vi "instr.DSO2002A.vi"(0 "VISA资源名称":refnum<visa-resource-name>, 1 "CMD":T2(ring), 2 "Trigger Mode":enum16{" TV", " GLITch", " EDGE", " PATTern"}(ring), 3 "Trigger Sweep":enum16{" AUTO", " NORMAL"}(ring), 4 "SignalFreq(kHz)":dbl=1.0, 5 "错误输入（无错误）":errorcluster, 6 "SignalVpp(V)":dbl=5.0, 7 "source":enum16{"  CHANnel1", "  CHANnel2"}(ring), 8 "Polarity":enum16{" NEGative", " POSitive"}(ring), 9 "Acquire Mode":enum16{" SEGMented", " RTIMe"}(ring), 10 "Standard":enum16{" PAL", " NTSC", " PALM", " SECam"}(ring), 11 "Reference":enum16{" CENTer", " LEFT", " RIGHt"}(ring), 13 "Acquire Type":T1(ring)) -> (14 "OK?":bool, 15 "Return Value":dbl, 18 "波形图":u8[](graph), 19 "错误输出":errorcluster)   [LabVIEW 2012, in "Lib_UEL.ATE.lvlib" / "Lib_Instrument.lvlib"]
uses:
  Lib_Instrument.lvlib
panel:
  in  "?":enum32{"TV", "Glitch"}(tab)
  in  "Setting":refnum<k24>(container)
  # "- 初始版本。\n- 2012-12-03: 增加获取图像命令，增加RESET命令。\n              命令子VI开放命令超时设置，默认超时为200mS。\n              留意：RESET命令需要1000mS超时才能正确工作。 \n-2013-5-20:增加触发&获取一部分功能\n-2013-5-21:增加自动获取和交流采集"
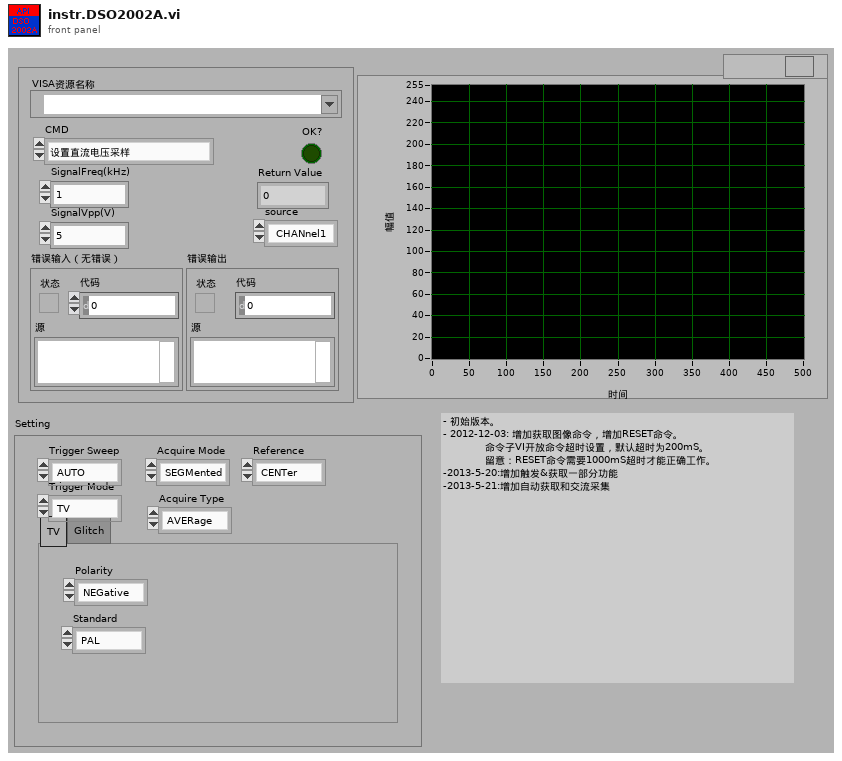
[diagram p1: front panel]
types:
  T1 = enum16{" AVERage", " NORMal", " HRESolution", " PEAK", ""}
  T2 = enum16{"设置直流电压采样", "设置交流电压采样", "获取直流电压值", "设置RMS采样", "获取RMS值", "设置频率采样", "获取频率值", "获取VPP", "重设Timing", "获取波形图", "RESET", "OFFSET", "设置触发模式", "设置获取模式", "自动获取", "Measure Vavg"}
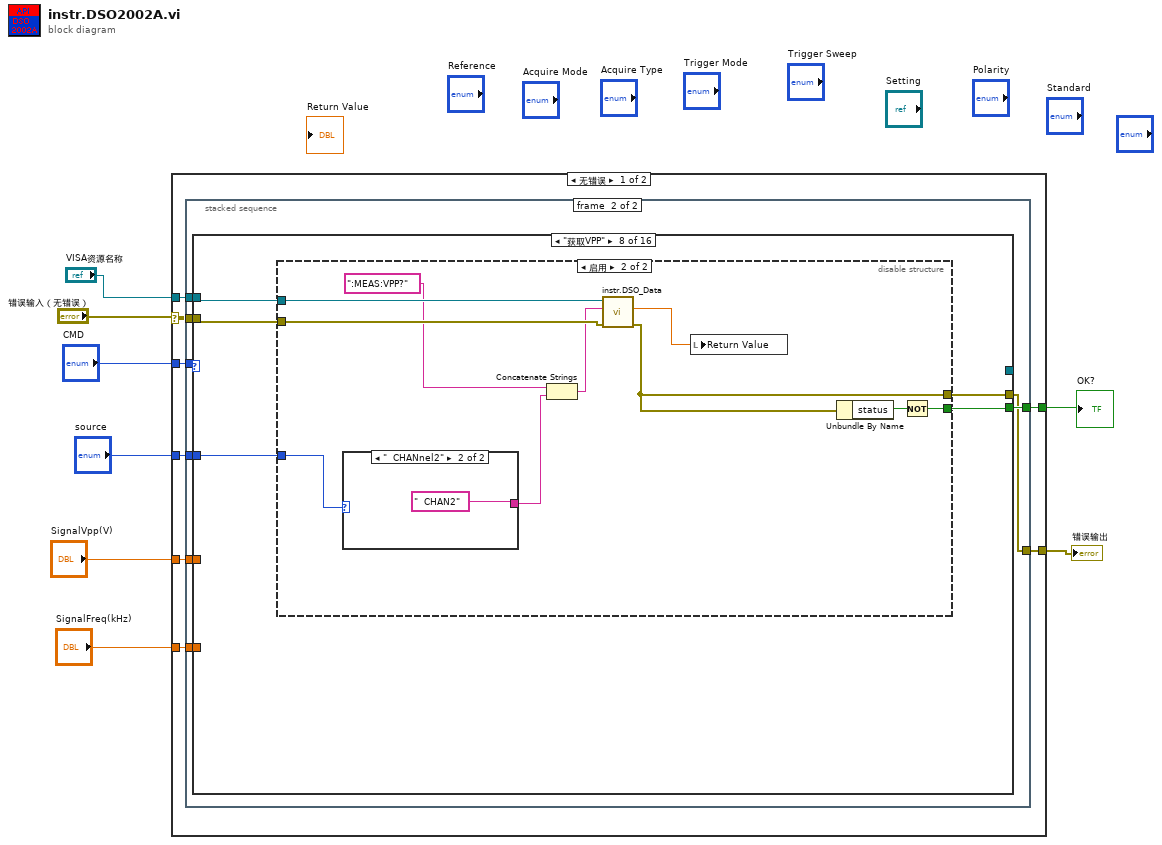
[diagram p0: block diagram]
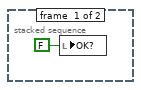
[diagram p2: hidden frame]
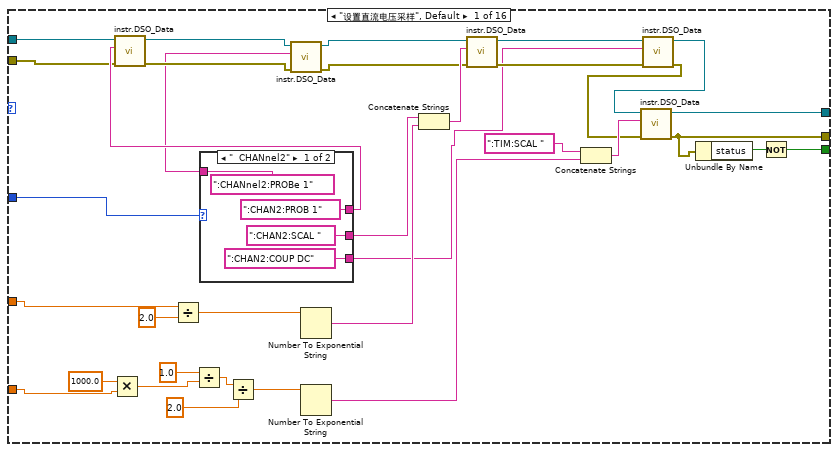
[diagram p3: hidden frame]
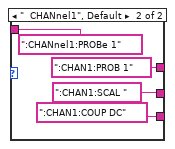
[diagram p4: hidden frame]
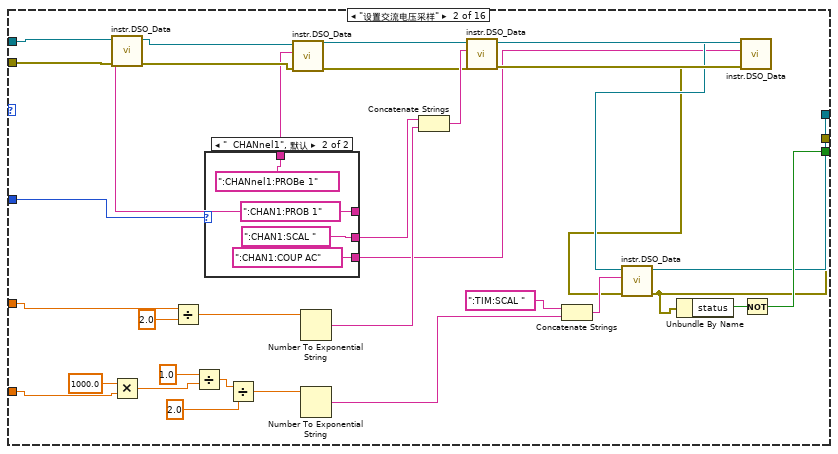
[diagram p5: hidden frame]
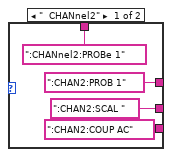
[diagram p6: hidden frame]
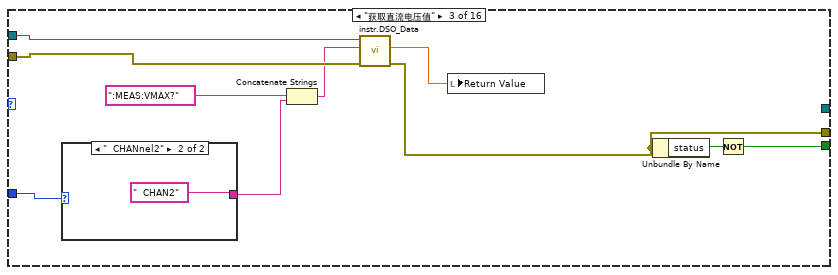
[diagram p7: hidden frame]
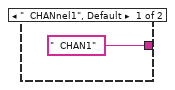
[diagram p8: hidden frame]
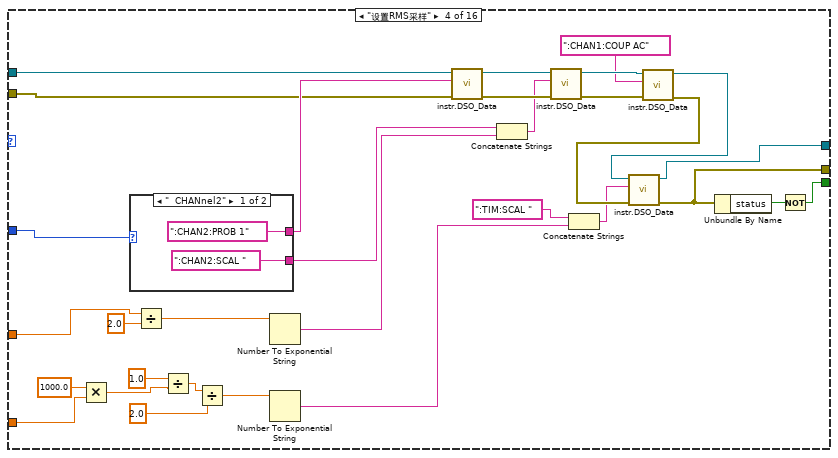
[diagram p9: hidden frame]
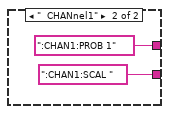
[diagram p10: hidden frame]
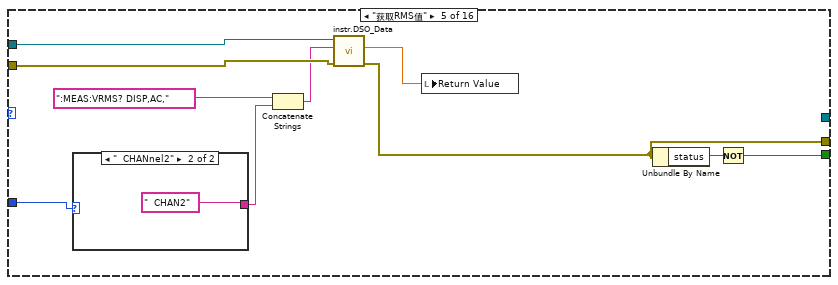
[diagram p11: hidden frame]
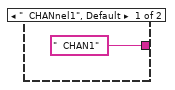
[diagram p12: hidden frame]
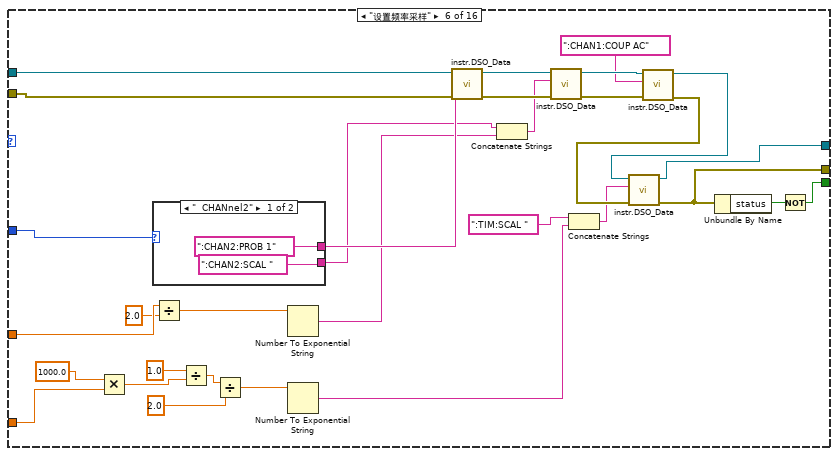
[diagram p13: hidden frame]
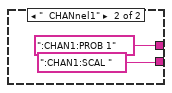
[diagram p14: hidden frame]
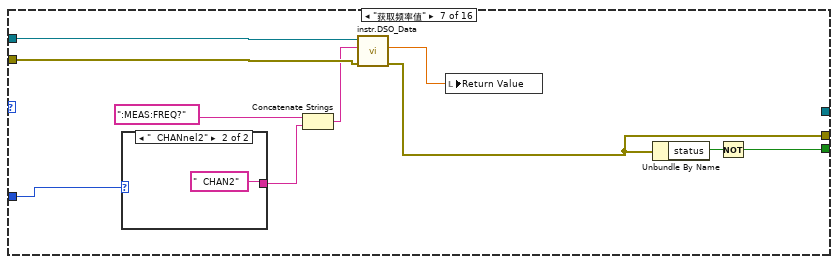
[diagram p15: hidden frame]
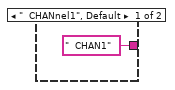
[diagram p16: hidden frame]
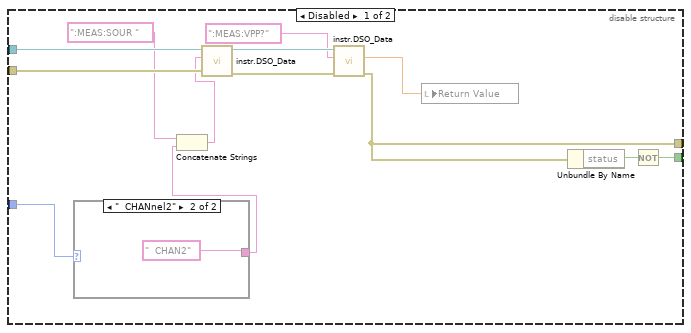
[diagram p17: hidden frame]
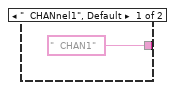
[diagram p18: hidden frame]
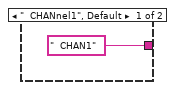
[diagram p19: hidden frame]
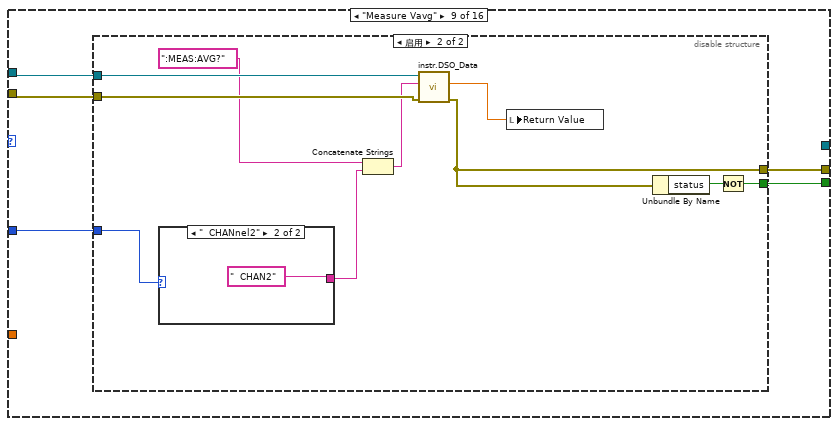
[diagram p20: hidden frame]
diagram:
  n1 = case shown="无错误" "错误输入（无错误）" {
    selector: "错误输入（无错误）" -> [w14 w428]
    tunnel: "VISA资源名称" -> [w16 _]
    tunnel: "CMD" -> [w15 _]
    tunnel: [w13 FALSE] -> w5
    tunnel: "SignalFreq(kHz)" -> [w12 _]
    tunnel: "SignalVpp(V)" -> [w11 _]
    tunnel: [w10 w428] -> w2
    tunnel: "source" -> [w9 _]
    frame No Error {
      n2 = stacked-sequence {
        tunnel: w16 -> [_ w25]
        tunnel: w15 -> [_ w24]
        tunnel: w14 -> [_ w18]
        tunnel: [_ w21] -> w13
        tunnel: w12 -> [_ w23]
        tunnel: w11 -> [_ w22]
        tunnel: [_ w20] -> w10
        tunnel: w9 -> [_ w19]
        frame #0 {
          n3 = local write "OK?"(FALSE ("OK?")) -> ()
        }
        frame #1 {
          n4 = case shown="\"获取VPP\"" w24 {
            tunnel: w25 -> [w34 w74 w119 w123 w166 w170 w213 w220 w252 w283 w306 w322 w361 w373 w420 w426]
            tunnel: [w56 w97 w115 w145 w162 w192 w209 w218 w250 w294 w310 w348 w356 w367 w403 w422] -> w21
            tunnel: w23 -> [w46 w87 _ w141 _ w188 _ _ _ w290 _ _ _ _ _ _]
            tunnel: w22 -> [w47 w88 _ w132 _ w179 _ _ _ _ _ _ _ w365 _ _]
            tunnel: [w38 w79 _ w125 _ w173 _ _ _ w281 w308 w327 w354 w371 w411 w424] -> _
            tunnel: [w37 w78 w114 w126 w161 w174 w208 w217 w249 w280 w307 w317 w353 w366 w402 w421] -> w20
            tunnel: w19 -> [w36 w77 w113 w124 w160 w172 w204 w216 w248 _ w304 _ _ _ _ _]
            tunnel: w18 -> [w33 w71 w118 w122 w165 w169 w212 w219 w251 w282 w305 w321 w360 w377 w419 w425]
            frame "设置直流电压采样", Default {
              n5 = Multiply(x=1000.0, y=w46) -> (x*y=w52:dbl)
              n6 = Divide(x=w47, y=2.0) -> (x/y=w48:dbl)
              n7 = Divide(x=1.0, y=w52) -> (x/y=w54:dbl)
              n8 = case shown="\"  CHANnel2\"" w36 {
                tunnel: [":CHAN2:PROB 1" ("CMD write") ":CHAN1:PROB 1" ("CMD write")] -> w59
                tunnel: [":CHAN2:SCAL " ("CMD write") ":CHAN1:SCAL " ("CMD write")] -> w35
                tunnel: [":CHAN2:COUP DC" ("CMD write") ":CHAN1:COUP DC" ("CMD write")] -> w32
                tunnel: [":CHANnel2:PROBe 1" ("CMD write") ":CHANnel1:PROBe 1" ("CMD write")] -> w26
                frame "  CHANnel2" {
                }
                frame "  CHANnel1", Default {
                }
              }
              n9 = call "instr.DSO_Data.vi"("错误输入（无错误）"=w33, "CMD write"=w59, "VISA.in"=w34) -> ("错误输出"=w28:errorcluster, "VISA.out"=w30:refnum<visa-resource-name>)  [unwired: 5 in, 2 out]
              n10 = Divide(x=w54, y=2.0) -> (x/y=w50:dbl)
              n11 = call "instr.DSO_Data.vi"("错误输入（无错误）"=w28, "CMD write"=w26, "VISA.in"=w30) -> ("错误输出"=w27:errorcluster, "VISA.out"=w29:refnum<visa-resource-name>)  [unwired: 5 in, 2 out]
              n12 = Number To Exponential String(number=w48) -> (E-format string=w40:string)  [unwired: 3 in]
              n13 = Number To Exponential String(number=w50) -> (E-format string=w41:string)  [unwired: 3 in]
              n14 = Concatenate Strings(w35, w40) -> (w39:string)
              n15 = call "instr.DSO_Data.vi"("错误输入（无错误）"=w27, "CMD write"=w39, "VISA.in"=w29) -> ("错误输出"=w58:errorcluster, "VISA.out"=w31:refnum<visa-resource-name>)  [unwired: 5 in, 2 out]
              n16 = Concatenate Strings(":TIM:SCAL " ("CMD write"), w41) -> (w44:string)
              n17 = call "instr.DSO_Data.vi"("错误输入（无错误）"=w58, "CMD write"=w32, "VISA.in"=w31) -> ("错误输出"=w42:errorcluster, "VISA.out"=w43:refnum<visa-resource-name>)  [unwired: 5 in, 2 out]
              n18 = call "instr.DSO_Data.vi"("错误输入（无错误）"=w42, "CMD write"=w44, "VISA.in"=w43) -> ("错误输出"=w37:errorcluster, "VISA.out"=w38:refnum<visa-resource-name>)  [unwired: 5 in, 2 out]
              n19 = Unbundle By Name(w37) -> ("status"=w57:bool)
              n20 = Not(x=w57) -> (.not. x?=w56:bool)
            }
            frame "设置交流电压采样" {
              n21 = Multiply(x=1000.0, y=w87) -> (x*y=w93:dbl)
              n22 = Divide(x=w88, y=2.0) -> (x/y=w89:dbl)
              n23 = Divide(x=1.0, y=w93) -> (x/y=w95:dbl)
              n24 = case shown="\"  CHANnel1\", 默认" w77 {
                tunnel: [":CHAN2:PROB 1" ("CMD write") ":CHAN1:PROB 1" ("CMD write")] -> w101
                tunnel: [":CHAN2:SCAL " ("CMD write") ":CHAN1:SCAL " ("CMD write")] -> w76
                tunnel: [":CHAN2:COUP AC" ("CMD write") ":CHAN1:COUP AC" ("CMD write")] -> w75
                tunnel: [":CHANnel2:PROBe 1" ("CMD write") ":CHANnel1:PROBe 1" ("CMD write")] -> w68
                frame "  CHANnel2" {
                }
                frame "  CHANnel1", Default {
                }
              }
              n25 = call "instr.DSO_Data.vi"("错误输入（无错误）"=w71, "CMD write"=w101, "VISA.in"=w74) -> ("错误输出"=w72:errorcluster, "VISA.out"=w73:refnum<visa-resource-name>)  [unwired: 5 in, 2 out]
              n26 = Divide(x=w95, y=2.0) -> (x/y=w91:dbl)
              n27 = call "instr.DSO_Data.vi"("错误输入（无错误）"=w72, "CMD write"=w68, "VISA.in"=w73) -> ("错误输出"=w70:errorcluster, "VISA.out"=w69:refnum<visa-resource-name>)  [unwired: 5 in, 2 out]
              n28 = Number To Exponential String(number=w89) -> (E-format string=w81:string)  [unwired: 3 in]
              n29 = Number To Exponential String(number=w91) -> (E-format string=w82:string)  [unwired: 3 in]
              n30 = Concatenate Strings(w76, w81) -> (w80:string)
              n31 = call "instr.DSO_Data.vi"("错误输入（无错误）"=w70, "CMD write"=w80, "VISA.in"=w69) -> ("错误输出"=w99:errorcluster, "VISA.out"=w100:refnum<visa-resource-name>)  [unwired: 5 in, 2 out]
              n32 = Concatenate Strings(":TIM:SCAL " ("CMD write"), w82) -> (w85:string)
              n33 = call "instr.DSO_Data.vi"("错误输入（无错误）"=w99, "CMD write"=w75, "VISA.in"=w100) -> ("错误输出"=w83:errorcluster, "VISA.out"=w84:refnum<visa-resource-name>)  [unwired: 5 in, 2 out]
              n34 = call "instr.DSO_Data.vi"("错误输入（无错误）"=w83, "CMD write"=w85, "VISA.in"=w84) -> ("错误输出"=w78:errorcluster, "VISA.out"=w79:refnum<visa-resource-name>)  [unwired: 5 in, 2 out]
              n35 = Unbundle By Name(w78) -> ("status"=w98:bool)
              n36 = Not(x=w98) -> (.not. x?=w97:bool)
            }
            frame "获取直流电压值" {
              n37 = case shown="\"  CHANnel2\"" w113 {
                tunnel: ["  CHAN1" ("CMD write") "  CHAN2" ("CMD write")] -> w111
                frame "  CHANnel1", Default {
                }
                frame "  CHANnel2" {
                }
              }
              n38 = Concatenate Strings(":MEAS:VMAX?" ("CMD write"), w111) -> (w110:string)
              n39 = call "instr.DSO_Data.vi"("错误输入（无错误）"=w118, "CMD write"=w110, "VISA.in"=w119) -> ("错误输出"=w114:errorcluster, "Value"=w117:dbl)  [unwired: 5 in, 2 out]
              n40 = local write "Return Value"(w117) -> ()
              n41 = Unbundle By Name(w114) -> ("status"=w116:bool)
              n42 = Not(x=w116) -> (.not. x?=w115:bool)
            }
            frame "设置RMS采样" {
              n43 = Multiply(x=1000.0, y=w141) -> (x*y=w140:dbl)
              n44 = case shown="\"  CHANnel2\"" w124 {
                tunnel: [":CHAN2:PROB 1" ("CMD write") ":CHAN1:PROB 1" ("CMD write")] -> w152
                tunnel: [":CHAN2:SCAL " ("CMD write") ":CHAN1:SCAL " ("CMD write")] -> w130
                frame "  CHANnel2" {
                }
                frame "  CHANnel1" {
                }
              }
              n45 = Divide(x=w132, y=2.0) -> (x/y=w129:dbl)
              n46 = Divide(x=1.0, y=w140) -> (x/y=w143:dbl)
              n47 = Divide(x=w143, y=2.0) -> (x/y=w138:dbl)
              n48 = Number To Exponential String(number=w129) -> (E-format string=w128:string)  [unwired: 3 in]
              n49 = Number To Exponential String(number=w138) -> (E-format string=w134:string)  [unwired: 3 in]
              n50 = call "instr.DSO_Data.vi"("错误输入（无错误）"=w122, "CMD write"=w152, "VISA.in"=w123) -> ("错误输出"=w150:errorcluster, "VISA.out"=w151:refnum<visa-resource-name>)  [unwired: 5 in, 2 out]
              n51 = Concatenate Strings(w130, w128) -> (w127:string)
              n52 = call "instr.DSO_Data.vi"("错误输入（无错误）"=w150, "CMD write"=w127, "VISA.in"=w151) -> ("错误输出"=w148:errorcluster, "VISA.out"=w149:refnum<visa-resource-name>)  [unwired: 5 in, 2 out]
              n53 = Concatenate Strings(":TIM:SCAL " ("CMD write"), w134) -> (w133:string)
              n54 = call "instr.DSO_Data.vi"("错误输入（无错误）"=w148, "CMD write"=":CHAN1:COUP AC", "VISA.in"=w149) -> ("错误输出"=w136:errorcluster, "VISA.out"=w137:refnum<visa-resource-name>)  [unwired: 5 in, 2 out]
              n55 = call "instr.DSO_Data.vi"("错误输入（无错误）"=w136, "CMD write"=w133, "VISA.in"=w137) -> ("错误输出"=w126:errorcluster, "VISA.out"=w125:refnum<visa-resource-name>)  [unwired: 5 in, 2 out]
              n56 = Unbundle By Name(w126) -> ("status"=w146:bool)
              n57 = Not(x=w146) -> (.not. x?=w145:bool)
            }
            frame "获取RMS值" {
              n58 = case shown="\"  CHANnel2\"" w160 {
                tunnel: ["  CHAN1" ("CMD write") "  CHAN2" ("CMD write")] -> w158
                frame "  CHANnel1", Default {
                }
                frame "  CHANnel2" {
                }
              }
              n59 = Concatenate Strings(":MEAS:VRMS? DISP,AC," ("CMD write"), w158) -> (w157:string)
              n60 = call "instr.DSO_Data.vi"("错误输入（无错误）"=w165, "CMD write"=w157, "VISA.in"=w166) -> ("错误输出"=w161:errorcluster, "Value"=w164:dbl)  [unwired: 5 in, 2 out]
              n61 = local write "Return Value"(w164) -> ()
              n62 = Unbundle By Name(w161) -> ("status"=w163:bool)
              n63 = Not(x=w163) -> (.not. x?=w162:bool)
            }
            frame "设置频率采样" {
              n64 = Multiply(x=1000.0, y=w188) -> (x*y=w187:dbl)
              n65 = case shown="\"  CHANnel2\"" w172 {
                tunnel: [":CHAN2:PROB 1" ("CMD write") ":CHAN1:PROB 1" ("CMD write")] -> w199
                tunnel: [":CHAN2:SCAL " ("CMD write") ":CHAN1:SCAL " ("CMD write")] -> w171
                frame "  CHANnel2" {
                }
                frame "  CHANnel1" {
                }
              }
              n66 = Divide(x=w179, y=2.0) -> (x/y=w177:dbl)
              n67 = Divide(x=1.0, y=w187) -> (x/y=w190:dbl)
              n68 = Divide(x=w190, y=2.0) -> (x/y=w185:dbl)
              n69 = Number To Exponential String(number=w177) -> (E-format string=w176:string)  [unwired: 3 in]
              n70 = Number To Exponential String(number=w185) -> (E-format string=w181:string)  [unwired: 3 in]
              n71 = call "instr.DSO_Data.vi"("错误输入（无错误）"=w169, "CMD write"=w199, "VISA.in"=w170) -> ("错误输出"=w197:errorcluster, "VISA.out"=w198:refnum<visa-resource-name>)  [unwired: 5 in, 2 out]
              n72 = Concatenate Strings(w171, w176) -> (w175:string)
              n73 = call "instr.DSO_Data.vi"("错误输入（无错误）"=w197, "CMD write"=w175, "VISA.in"=w198) -> ("错误输出"=w195:errorcluster, "VISA.out"=w196:refnum<visa-resource-name>)  [unwired: 5 in, 2 out]
              n74 = Concatenate Strings(":TIM:SCAL " ("CMD write"), w181) -> (w180:string)
              n75 = call "instr.DSO_Data.vi"("错误输入（无错误）"=w195, "CMD write"=":CHAN1:COUP AC", "VISA.in"=w196) -> ("错误输出"=w183:errorcluster, "VISA.out"=w184:refnum<visa-resource-name>)  [unwired: 5 in, 2 out]
              n76 = call "instr.DSO_Data.vi"("错误输入（无错误）"=w183, "CMD write"=w180, "VISA.in"=w184) -> ("错误输出"=w174:errorcluster, "VISA.out"=w173:refnum<visa-resource-name>)  [unwired: 5 in, 2 out]
              n77 = Unbundle By Name(w174) -> ("status"=w193:bool)
              n78 = Not(x=w193) -> (.not. x?=w192:bool)
            }
            frame "获取频率值" {
              n79 = case shown="\"  CHANnel2\"" w204 {
                tunnel: ["  CHAN1" ("CMD write") "  CHAN2" ("CMD write")] -> w206
                frame "  CHANnel1", Default {
                }
                frame "  CHANnel2" {
                }
              }
              n80 = Concatenate Strings(":MEAS:FREQ?" ("CMD write"), w206) -> (w205:string)
              n81 = call "instr.DSO_Data.vi"("错误输入（无错误）"=w212, "CMD write"=w205, "VISA.in"=w213) -> ("错误输出"=w208:errorcluster, "Value"=w211:dbl)  [unwired: 5 in, 2 out]
              n82 = local write "Return Value"(w211) -> ()
              n83 = Unbundle By Name(w208) -> ("status"=w210:bool)
              n84 = Not(x=w210) -> (.not. x?=w209:bool)
            }
            frame "获取VPP" {
              n85 = disable-structure shown="启用" {
                disable-tunnel: w220 -> [w228 w245]
                disable-tunnel: w219 -> [w227 w244]
                disable-tunnel: [w231 w241] -> w218
                disable-tunnel: [w230 w240] -> w217
                disable-tunnel: w216 -> [w229 w239]
                frame Disabled {
                  n86 = case shown="\"  CHANnel2\"" w229 {
                    tunnel: ["  CHAN1" ("CMD write") "  CHAN2" ("CMD write")] -> w222
                    frame "  CHANnel1", Default {
                    }
                    frame "  CHANnel2" {
                    }
                  }
                  n87 = Concatenate Strings(":MEAS:SOUR " ("CMD write"), w222) -> (w221:string)
                  n88 = call "instr.DSO_Data.vi"("错误输入（无错误）"=w227, "CMD write"=w221, "VISA.in"=w228) -> ("错误输出"=w225:errorcluster, "VISA.out"=w226:refnum<visa-resource-name>)  [unwired: 5 in, 2 out]
                  n89 = call "instr.DSO_Data.vi"("错误输入（无错误）"=w225, "CMD write"=":MEAS:VPP?", "VISA.in"=w226) -> ("错误输出"=w230:errorcluster, "Value"=w233:dbl)  [unwired: 5 in, 2 out]
                  n90 = local write "Return Value"(w233) -> ()
                  n91 = Unbundle By Name(w230) -> ("status"=w232:bool)
                  n92 = Not(x=w232) -> (.not. x?=w231:bool)
                }
                frame Enabled {
                  n93 = case shown="\"  CHANnel2\"" w239 {
                    tunnel: ["  CHAN1" ("CMD write") "  CHAN2" ("CMD write")] -> w238
                    frame "  CHANnel1", Default {
                    }
                    frame "  CHANnel2" {
                    }
                  }
                  n94 = Concatenate Strings(":MEAS:VPP?" ("CMD write"), w238) -> (w236:string)
                  n95 = call "instr.DSO_Data.vi"("错误输入（无错误）"=w244, "CMD write"=w236, "VISA.in"=w245) -> ("错误输出"=w240:errorcluster, "Value"=w243:dbl)  [unwired: 5 in, 2 out]
                  n96 = local write "Return Value"(w243) -> ()
                  n97 = Unbundle By Name(w240) -> ("status"=w242:bool)
                  n98 = Not(x=w242) -> (.not. x?=w241:bool)
                }
              }
            }
            frame "Measure Vavg" {
              n99 = disable-structure shown="启用" {
                disable-tunnel: w252 -> [w260 w277]
                disable-tunnel: w251 -> [w259 w276]
                disable-tunnel: [w263 w273] -> w250
                disable-tunnel: [w262 w272] -> w249
                disable-tunnel: w248 -> [w261 w271]
                frame Disabled {
                  n100 = case shown="\"  CHANnel2\"" w261 {
                    tunnel: ["  CHAN1" ("CMD write") "  CHAN2" ("CMD write")] -> w254
                    frame "  CHANnel1", Default {
                    }
                    frame "  CHANnel2" {
                    }
                  }
                  n101 = Concatenate Strings(":MEAS:SOUR " ("CMD write"), w254) -> (w253:string)
                  n102 = call "instr.DSO_Data.vi"("错误输入（无错误）"=w259, "CMD write"=w253, "VISA.in"=w260) -> ("错误输出"=w257:errorcluster, "VISA.out"=w258:refnum<visa-resource-name>)  [unwired: 5 in, 2 out]
                  n103 = call "instr.DSO_Data.vi"("错误输入（无错误）"=w257, "CMD write"=":MEAS:VPP?", "VISA.in"=w258) -> ("错误输出"=w262:errorcluster, "Value"=w265:dbl)  [unwired: 5 in, 2 out]
                  n104 = local write "Return Value"(w265) -> ()
                  n105 = Unbundle By Name(w262) -> ("status"=w264:bool)
                  n106 = Not(x=w264) -> (.not. x?=w263:bool)
                }
                frame Enabled {
                  n107 = case shown="\"  CHANnel2\"" w271 {
                    tunnel: ["  CHAN1" ("CMD write") "  CHAN2" ("CMD write")] -> w270
                    frame "  CHANnel1", Default {
                    }
                    frame "  CHANnel2" {
                    }
                  }
                  n108 = Concatenate Strings(":MEAS:AVG?" ("CMD write"), w270) -> (w268:string)
                  n109 = call "instr.DSO_Data.vi"("错误输入（无错误）"=w276, "CMD write"=w268, "VISA.in"=w277) -> ("错误输出"=w272:errorcluster, "Value"=w275:dbl)  [unwired: 5 in, 2 out]
                  n110 = local write "Return Value"(w275) -> ()
                  n111 = Unbundle By Name(w272) -> ("status"=w274:bool)
                  n112 = Not(x=w274) -> (.not. x?=w273:bool)
                }
              }
            }
            frame "重设Timing" {
              n113 = Multiply(x=1000.0, y=w290) -> (x*y=w289:dbl)
              n114 = Divide(x=1.0, y=w289) -> (x/y=w292:dbl)
              n115 = Divide(x=w292, y=2.0) -> (x/y=w287:dbl)
              n116 = Number To Exponential String(number=w287) -> (E-format string=w285:string)  [unwired: 3 in]
              n117 = Concatenate Strings(":TIM:SCAL " ("CMD write"), w285) -> (w284:string)
              n118 = call "instr.DSO_Data.vi"("错误输入（无错误）"=w282, "CMD write"=w284, "VISA.in"=w283) -> ("错误输出"=w280:errorcluster, "VISA.out"=w281:refnum<visa-resource-name>)  [unwired: 5 in, 2 out]
              n119 = Unbundle By Name(w280) -> ("status"=w295:bool)
              n120 = Not(x=w295) -> (.not. x?=w294:bool)
            }
            frame "OFFSET" {
              # "设置零点光标到屏幕底部，从底部开始0.5格的位置"
              n121 = case shown="\"  CHANnel2\"" w304 {
                tunnel: [":CHAN2:SCAL?" ("CMD write") ":CHAN1:SCAL?" ("CMD write")] -> w303
                frame "  CHANnel2" {
                }
                frame "  CHANnel1" {
                }
              }
              n122 = case shown="\"  CHANnel2\"" w304 {
                tunnel: [":CHAN2:OFFS " ("CMD write") ":CHAN1:OFFS " ("CMD write")] -> w298
                frame "  CHANnel2" {
                }
                frame "  CHANnel1" {
                }
              }
              n123 = call "instr.DSO_Data.vi"("错误输入（无错误）"=w305, "CMD write"=w303, "VISA.in"=w306) -> ("错误输出"=w296:errorcluster, "Value"=w302:dbl, "VISA.out"=w297:refnum<visa-resource-name>)  [unwired: 5 in, 1 out]
              n124 = Multiply(x=w302, y=3.5) -> (x*y=w300:dbl)
              n125 = Number To Fractional String(number=w300) -> (F-format string=w299:string)  [unwired: 3 in]
              n126 = Concatenate Strings(w298, w299) -> (w309:string)
              n127 = call "instr.DSO_Data.vi"("错误输入（无错误）"=w296, "CMD write"=w309, "VISA.in"=w297) -> ("错误输出"=w307:errorcluster, "VISA.out"=w308:refnum<visa-resource-name>)  [unwired: 5 in, 2 out]
              n128 = Unbundle By Name(w307) -> ("status"=w311:bool)
              n129 = Not(x=w311) -> (.not. x?=w310:bool)
            }
            frame "获取波形图" {
              w316 = u32 200 ("Timeout(ms)")
              w331 = ":WAVeform:"
              n130 = flat-sequence {
                tunnel: [w351] -> w330
                tunnel: w322 -> [w351]
                tunnel: [w350] -> w329
                tunnel: w321 -> [w350]
                frame #0 {
                }
              }
              n131 = Concatenate Strings(w331, "FORMat", "  BYTE" ("字符串")) -> (w336:string)
              n132 = property on="source" class="Enum (严格)"() -> ("RingText.Text"=w324:string)  [unwired: 2 in, 2 out]
              n133 = call "instr.DSO_Data.vi"("Timeout(ms)"=w316, "错误输入（无错误）"=w329, "CMD write"=w336, "VISA.in"=w330) -> ("错误输出"=w341:errorcluster, "VISA.out"=w342:refnum<visa-resource-name>)  [unwired: 4 in, 2 out]
              n134 = Concatenate Strings(w331, "SOURce", w324) -> (w344:string)
              n135 = call "instr.DSO_Data.vi"("Timeout(ms)"=w316, "错误输入（无错误）"=w341, "CMD write"=w344, "VISA.in"=w342) -> ("错误输出"=w339:errorcluster, "VISA.out"=w340:refnum<visa-resource-name>)  [unwired: 4 in, 2 out]
              n136 = Concatenate Strings(w331, "POINts", " 1000" ("字符串")) -> (w343:string)
              n137 = call "instr.DSO_Data.vi"("Timeout(ms)"=w316, "错误输入（无错误）"=w339, "CMD write"=w343, "VISA.in"=w340) -> ("错误输出"=w337:errorcluster, "VISA.out"=w338:refnum<visa-resource-name>)  [unwired: 4 in, 2 out]
              n138 = call "instr.DSO_Data.vi"("错误输入（无错误）"=w337, "CMD write"=":WAVeform:DATA?", "VISA.in"=w338) -> ("错误输出"=w318:errorcluster, "Reply info"=w326:string, "Value"=w319:dbl, "VISA.out"=w327:refnum<visa-resource-name>)  [unwired: 5 in]
              n139 = String To Byte Array(string=w326) -> (unsigned byte array=w320:u8[])
              n140 = flat-sequence {
                tunnel: [w349] -> w317
                tunnel: w318 -> [w349]
                frame #0 {
                }
              }
              n141 = Array Subset(array=w320, index=10 ("索引"), length=1000 ("长度")) -> (→"波形图":u8[])
              n142 = local write "Return Value"(w319) -> ()
              n143 = Unbundle By Name(w318) -> ("status"=w325:bool)
              n144 = Not(x=w325) -> (.not. x?=w348:bool)
            }
            frame "RESET" {
              n145 = call "instr.DSO_Data.vi"("Timeout(ms)"=u32 800, "错误输入（无错误）"=w360, "CMD write"="*RST", "VISA.in"=w361) -> ("错误输出"=w357:errorcluster, "VISA.out"=w358:refnum<visa-resource-name>)  [unwired: 4 in, 2 out]
              n146 = flat-sequence {
                tunnel: [w363] -> w354
                tunnel: w358 -> [w363]
                tunnel: [w362] -> w353
                tunnel: w357 -> [w362]
                frame #0 {
                  n147 = Wait (ms)(milliseconds to wait=u32 50 ("等待时间（毫秒）")) -> ()  [unwired: 1 out]
                }
              }
              n148 = Unbundle By Name(w353) -> ("status"=w352:bool)
              n149 = Not(x=w352) -> (.not. x?=w356:bool)
            }
            frame "设置触发模式" {
              n150 = property on="Trigger Sweep" class="Enum (严格)"() -> ("RingText.Text"=w370:string)  [unwired: 2 in, 2 out]
              n151 = local read "Trigger Mode"() -> (w376:enum16{" TV", " GLITch", " EDGE", " PATTern"})
              n152 = Concatenate Strings(":TRIGger:SWEep" ("字符串"), w370) -> (w375:string)
              n153 = call "instr.DSO_Data.vi"("错误输入（无错误）"=w377, "CMD write"=w375, "VISA.in"=w373) -> ("错误输出"=w369:errorcluster, "VISA.out"=w372:refnum<visa-resource-name>)  [unwired: 5 in, 2 out]
              n154 = case shown="\" EDGE\"" w376 {
                tunnel: w372 -> [w382 _ w401 _]
                tunnel: [w384 _ w398 _] -> w366
                tunnel: [w383 _ w400 _] -> w371
                tunnel: w369 -> [w380 _ w399 _]
                tunnel: w365 -> [_ _ w397 _]
                frame " TV", Default {
                  n155 = property on="Standard" class="Enum (严格)"() -> ("RingText.Text"=w390:string)  [unwired: 2 in, 2 out]
                  n156 = property on="Polarity" class="Enum (严格)"() -> ("RingText.Text"=w389:string)  [unwired: 2 in, 2 out]
                  n157 = Concatenate Strings(":TRIGger:TV:POLarity", w389) -> (w392:string)
                  n158 = Concatenate Strings(":TRIGger:TV:STANdard" ("字符串"), w390) -> (w391:string)
                  n159 = call "instr.DSO_Data.vi"("错误输入（无错误）"=w380, "CMD write"=":TRIGger:MODE TV" ("字符串"), "VISA.in"=w382) -> ("错误输出"=w378:errorcluster, "VISA.out"=w381:refnum<visa-resource-name>)  [unwired: 5 in, 2 out]
                  n160 = call "instr.DSO_Data.vi"("错误输入（无错误）"=w378, "CMD write"=w392, "VISA.in"=w381) -> ("错误输出"=w385:errorcluster, "VISA.out"=w386:refnum<visa-resource-name>)  [unwired: 5 in, 2 out]
                  n161 = call "instr.DSO_Data.vi"("错误输入（无错误）"=w385, "CMD write"=w391, "VISA.in"=w386) -> ("错误输出"=w384:errorcluster, "VISA.out"=w383:refnum<visa-resource-name>)  [unwired: 5 in, 2 out]
                }
                frame " GLITch" {
                }
                frame " EDGE" {
                  n162 = Number To Fractional String(number=w397, precision (6)=i16 2 ("精度(6)")) -> (F-format string=w395:string)  [unwired: 2 in]
                  n163 = Concatenate Strings(":TRIGger:LEV " ("字符串"), w395) -> (w394:string)
                  n164 = call "instr.DSO_Data.vi"("错误输入（无错误）"=w399, "CMD write"=w394, "VISA.in"=w401) -> ("错误输出"=w398:errorcluster, "VISA.out"=w400:refnum<visa-resource-name>)  [unwired: 5 in, 2 out]
                }
                frame " PATTern" {
                }
              }
              n165 = Unbundle By Name(w366) -> ("status"=w368:bool)
              n166 = Not(x=w368) -> (.not. x?=w367:bool)
            }
            frame "设置获取模式" {
              n167 = property on="Reference" class="Enum (严格)"() -> ("RingText.Text"=w417:string)  [unwired: 2 in, 2 out]
              n168 = Concatenate Strings(":TIMEebase:REFerence" ("字符串"), w417) -> (w416:string)
              n169 = call "instr.DSO_Data.vi"("错误输入（无错误）"=w419, "CMD write"=w416, "VISA.in"=w420) -> ("错误输出"=w413:errorcluster, "VISA.out"=w415:refnum<visa-resource-name>)  [unwired: 5 in, 2 out]
              n170 = property on="Acquire Mode" class="Enum (严格)"() -> ("RingText.Text"=w409:string)  [unwired: 2 in, 2 out]
              n171 = Concatenate Strings(":ACQuire:MODE" ("字符串"), w409) -> (w408:string)
              n172 = call "instr.DSO_Data.vi"("错误输入（无错误）"=w413, "CMD write"=w408, "VISA.in"=w415) -> ("错误输出"=w412:errorcluster, "VISA.out"=w414:refnum<visa-resource-name>)  [unwired: 5 in, 2 out]
              n173 = property on="Acquire Type" class="Enum (严格)"() -> ("RingText.Text"=w406:string)  [unwired: 2 in, 2 out]
              n174 = Concatenate Strings(":ACQuire:TYPE" ("字符串"), w406) -> (w405:string)
              n175 = call "instr.DSO_Data.vi"("错误输入（无错误）"=w412, "CMD write"=w405, "VISA.in"=w414) -> ("错误输出"=w402:errorcluster, "VISA.out"=w411:refnum<visa-resource-name>)  [unwired: 5 in, 2 out]
              n176 = Unbundle By Name(w402) -> ("status"=w404:bool)
              n177 = Not(x=w404) -> (.not. x?=w403:bool)
            }
            frame "自动获取" {
              n178 = call "instr.DSO_Data.vi"("错误输入（无错误）"=w425, "CMD write"=":AUToscale", "VISA.in"=w426) -> ("错误输出"=w421:errorcluster, "VISA.out"=w424:refnum<visa-resource-name>)  [unwired: 5 in, 2 out]
              n179 = Unbundle By Name(w421) -> ("status"=w423:bool)
              n180 = Not(x=w423) -> (.not. x?=w422:bool)
            }
          }
        }
      }
    }
    frame Error {
    }
  }
  "错误输出" <- w2
  "OK?" <- w5
